vi "UDP Sender.vi"() -> ()   [LabVIEW 2010]
doc: "This VI is designed to be used with the UDP Receiver VI. Run the UDP Receiver.vi first.\n\nThe UDP protocol differs from TCP in that there is no error-checking with the packets of information that are sent, and thus no guarantee whatsoever that an intended recipient will actually receive a given piece of data.\n\nUDP does offer the ability to \"broadcast\" data across a network--simply specify an IP Address of all ones (255.255.255.255) to attempt to broadcast information network-wide. Keep in mind that routers and other network hardware will generally refuse to forward the broadcast beyond certain points, so the extent of the broadcast will in practice be limited."
uses:
  6-OCU Neurons/6.1-UDP Saitek.ctl
panel:
  in  "s":bool
  in  "Cluster":T1 {"T-B" scale=-2147483648.0..2147483647.0; "T-A" scale=-2147483648.0..2147483647.0; "Y" scale=-2147483648.0..2147483647.0; "R" scale=-2147483648.0..2147483647.0; "P" scale=-2147483648.0..2147483647.0}
  out "type string":i16[](array[numeric])
  in  "# Repetitions":i32=10
  in  "Remote Port":u16=1337
  in  "Local Port":u16=1337
  in  "Remote Host":string="localhost"
  in  "Data String":string="<data>"
  in  "broadcast":bool
  # "Instructions:\n1. Open the UDP Receiver.vi located in the same library.\n2. Make sure that the Remote Port in this VI and the Port in the UDP Receive.vi are the same.\n3. Press the button if you want to broadcast the data to all the network, instead of sending it to a specific address.\n4. Change the number of times you want to send the data to the receiver in the # of Repetitions control.\n5. Follow the instructions on it's front panel.\nNote: This VI is built to work with the UDP Receiver.vi."
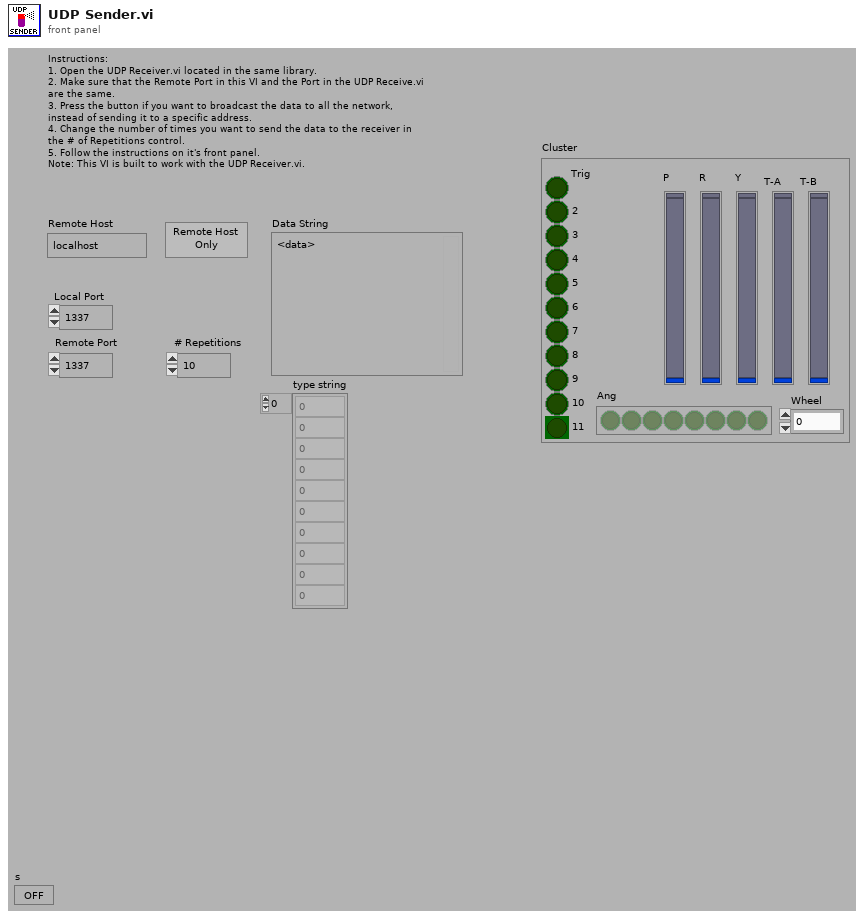
[diagram p1: front panel]
types:
  T1 = typedef "6.1-UDP Saitek.ctl" = cluster{"3":bool, "2":bool, "5":bool, "4":bool, "P":i32, "R":i32, "Y":i32, "T-A":i32, "T-B":i32, "7":bool, "6":bool, "9":bool, "8":bool, "Trig":bool, "Wheel":dbl, "Ang":bool[], "10":bool, "11":bool}
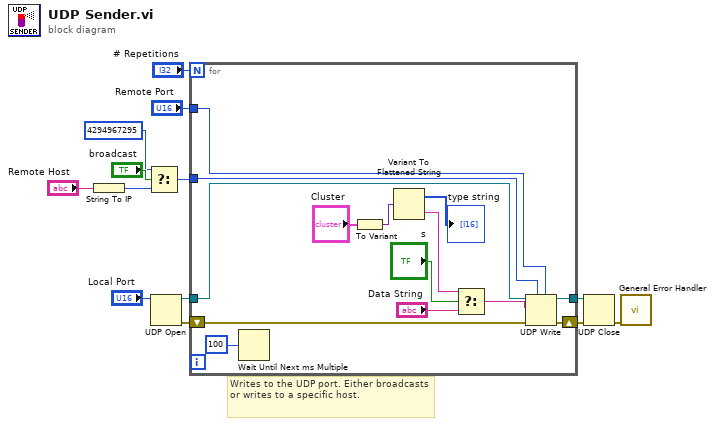
[diagram p0: block diagram]
diagram:
  # "Writes to the UDP port. Either broadcasts or writes to a specific host."
  n1 = String To IP(1:"Remote Host") -> (0:w5:u32)
  n2 = Select(t=u32 4294967295, s="broadcast", f=w5) -> (s? t:f=w4:u32)
  n3 = UDP Open(11:"Local Port") -> (port=w13:refnum<k16>, 0:w11:errorcluster)  [unwired: 1 in, 4 out]
  n4 = for {
    N: "# Repetitions" -> [_]
    tunnel: w13 -> [w25]
    tunnel: w4 -> [w27]
    tunnel: "Remote Port" -> [w26]
    shift-right: [w23] -> w10
    shift-left: w11 -> [w24]
    tunnel: [w22] -> w9
    n5 = Wait Until Next ms Multiple(millisecond multiple=u32 100) -> ()  [unwired: 1 out]
    n6 = To Variant(anything="Cluster") -> (Variant=w19:variant)
    n7 = Variant To Flattened String(Variant=w19) -> (data string=w18:string, 1:→"type string":i16[])
    n8 = Select(t=w18, s="s", f="Data String") -> (s? t:f=w17:string)
    n9 = UDP Write(address=w27, port or service name=w26, connection ID=w25, data in=w17, 8:w24) -> (error out=w23:errorcluster, 3:w22:refnum<k16>)  [unwired: 1 out]
  }
  n10 = UDP Close(connection ID=w9, 8:w10) -> (error out=w8:errorcluster)  [unwired: 1 out]
  n11 = call <vilib>:"General Error Handler.vi"("error in (no error)"=w8) -> ()  [unwired: 1 in, 14 out]
